vi "Defer Panel Updates.vi"(8 "error in (no error)":errorcluster, 10 "Defer?":bool, 11 "VI in":refnum<vi>) -> (0 "error out":errorcluster)   [LabVIEW 2016]
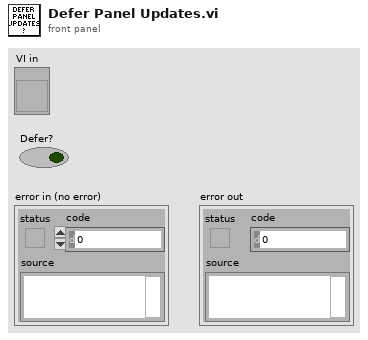
[diagram p1: front panel]
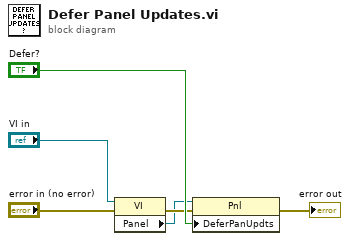
[diagram p0: block diagram]
diagram:
  n1 = property class="VI"(reference="VI in", error in="error in (no error)") -> (error out=w4:errorcluster, "Panel"=w1:refnum<vi>)  [unwired: 1 out]
  n2 = property class="Pnl"(reference=w1, error in=w4, "DeferPanUpdts"="Defer?") -> (error out=→"error out":errorcluster)  [unwired: 1 out]
